vi "Internal Open.vi"(0 "navX Device":T8={"Interface"={"Protocol"=enum."SERIAL", "Update Rate (4Hz-60Hz)"=4, "navX Open TypeDef"=variant}, "Notify Packet"=refnum, "Loop VI Refnum"=refnum} {"Interface"."Update Rate (4Hz-60Hz)" min=4 max=60 step=1}) -> (1 "Interface TypeDefs":T1 {"I2CDevRef"."Device Address" format="%.0x"}, 2 "error out":errorcluster)   [LabVIEW 2014, in "navX Library v2.lvlib"]
uses:
  navX Library v2.lvlib
  TypeDefs/navX Device TypeDef.ctl
  TypeDefs/navX Protocol TypeDef.ctl
  TypeDefs/navX Notify Packet TypeDef.ctl
  TypeDefs/navX Action TypeDef.ctl
  TypeDefs/navX Interface TypeDef.ctl
  <vilib>/Rock Robotics/WPI/SerialPort/WPI_SerialPortRef.ctl
  <vilib>/Rock Robotics/WPI/I2C/WPI_I2CDevRef.ctl
  <vilib>/Rock Robotics/SystemInterfaces/Typedef/FPGA_TypedefDigitalModule.ctl
  <vilib>/Rock Robotics/SystemInterfaces/i2clib/i2c_bus.ctl
  <vilib>/Rock Robotics/WPI/SPI/WPI_SPIDevRef.ctl
  <vilib>/Rock Robotics/SystemInterfaces/spilib/spi_bus.ctl
  TypeDefs/navX Open TypeDefs/navX Serial Open TypeDef.ctl
  NI WPI/WPI_SerialPort_USB.ctl
  TypeDefs/navX Open TypeDefs/navX I2C Open TypeDef.ctl
  TypeDefs/navX Open TypeDefs/navX SPI Open TypeDef.ctl
  NI WPI/NI WPI Serial USB.lvlib
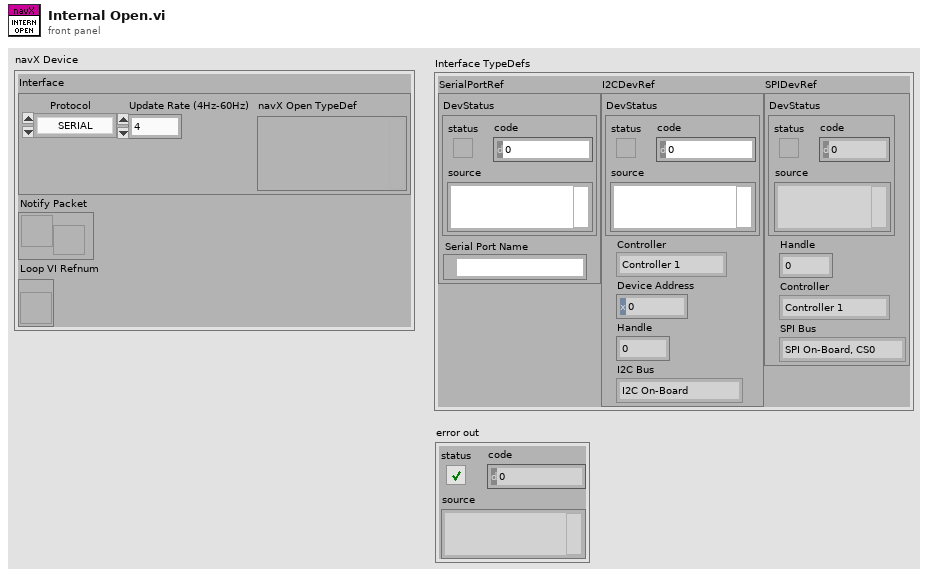
[diagram p1: front panel]
types:
  T1 = typedef "navX Library v2.lvlib/navX Interface TypeDef.ctl" = cluster{"SerialPortRef":T2, "I2CDevRef":T3, "SPIDevRef":T6}
  T2 = typedef "WPI_SerialPortRef.ctl" = cluster{"DevStatus":errorcluster, "Serial Port Name":refnum<visa-resource-name>}
  T3 = typedef "WPI_I2CDevRef.ctl" = cluster{"DevStatus":errorcluster, "Controller":T4, "Device Address":u8, "Handle":i32, "I2C Bus":T5}
  T4 = typedef "FPGA_TypedefDigitalModule.ctl" = enum16{"Controller 1"}
  T5 = typedef "i2c_bus.ctl" = enum16{"I2C On-Board", "I2C MXP", "Invalid"}
  T6 = typedef "WPI_SPIDevRef.ctl" = cluster{"DevStatus":errorcluster, "Handle":i32, "Controller":T4, "SPI Bus":T7}
  T7 = typedef "spi_bus.ctl" = enum16{"SPI On-Board, CS0", "SPI On-Board, CS1", "SPI On-Board, CS2", "SPI On-Board, CS3", "SPI MXP", "Invalid"}
  T8 = typedef "navX Library v2.lvlib/navX Device TypeDef.ctl" = cluster{"Interface":cluster{"Protocol":T9, "Update Rate (4Hz-60Hz)":u8, "navX Open TypeDef":variant}, "Notify Packet":refnum<notifier>, "Loop VI Refnum":refnum<vi>}
  T9 = typedef "navX Library v2.lvlib/navX Protocol TypeDef.ctl" = enum16{"SERIAL", "I2C", "SPI"}
  T10 = typedef "navX Library v2.lvlib/navX Serial Open TypeDef.ctl" = cluster{"Serial Port":T11, "Raw Data":bool}
  T11 = typedef "NI WPI Serial USB.lvlib/WPI_SerialPort_USB.ctl" = enum16{"Onboard RS-232", "MXP TTL", "USB"}
  T12 = typedef "navX Library v2.lvlib/navX I2C Open TypeDef.ctl" = cluster{"I2C Bus":T5}
  T13 = typedef "navX Library v2.lvlib/navX SPI Open TypeDef.ctl" = cluster{"SPI Bus":T7}
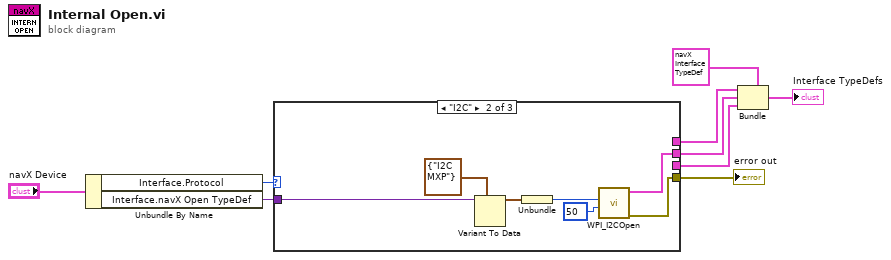
[diagram p0: block diagram]
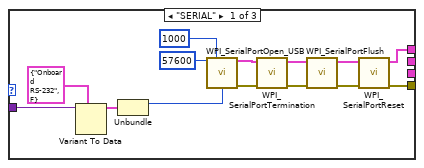
[diagram p2: hidden frame]
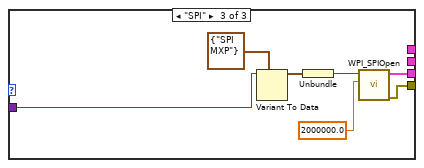
[diagram p3: hidden frame]
diagram:
  n1 = Unbundle By Name("navX Device") -> ("Interface.Protocol"=w5:T9, "Interface.navX Open TypeDef"=w4:variant)
  n2 = case shown="\"I2C\"" w5 {
    tunnel: w4 -> [w23 w29 w36]
    tunnel: [w11 _ _] -> w9
    tunnel: [w10 w25 w32] -> w3
    tunnel: [_ w24 _] -> w8
    tunnel: [_ _ w31] -> w7
    frame "SERIAL" {
      n3 = Variant To Data(type=T10 {"Serial Port"=enum."Onboard RS-232", "Raw Data"=FALSE} ("navX Serial Open"), Variant=w23) -> (data=w21:T10)  [unwired: 1 in, 1 out]
      n4 = Unbundle(w21) -> ("Serial Port"=w20:T11)  [unwired: 1 out]
      n5 = call "WPI_SerialPortOpen_USB.vi"("Baud Rate"=u32 57600, "Timeout Value (ms)"=u32 1000, "Serial Port"=w20) -> ("SerialPortRef"=w13:T2, "error out"=w12:errorcluster)  [unwired: 11 in]
      n6 = call <vilib>:"WPI_SerialPortTermination.vi"("error in (no error)"=w12, "SerialPortRef"=w13) -> ("error out"=w17:errorcluster, "SerialPortRef"=w16:T2)  [unwired: 8 in]
      n7 = call <vilib>:"WPI_SerialPortFlush.vi"("error in (no error)"=w17, "SerialPortRef"=w16) -> ("error out"=w14:errorcluster, "SerialPortRef"=w15:T2)  [unwired: 8 in]
      n8 = call <vilib>:"WPI_SerialPortReset.vi"("error in (no error)"=w14, "SerialPortRef"=w15) -> ("error out"=w10:errorcluster, "SerialPortRef"=w11:T2)  [unwired: 8 in]
    }
    frame "I2C" {
      n9 = Variant To Data(type=T12 {"I2C Bus"=enum."I2C MXP"} ("navX I2C Open"), Variant=w29) -> (data=w30:T12)  [unwired: 1 in, 1 out]
      n10 = Unbundle(w30) -> ("I2C Bus"=w27:T5)
      n11 = call <vilib>:"WPI_I2COpen.vi"("Device Address"=u8 50, "I2C Bus"=w27) -> ("error out"=w25:errorcluster, "I2CDevRef"=w24:T3)  [unwired: 8 in]
    }
    frame "SPI" {
      n12 = Variant To Data(type=T13 {"SPI Bus"=enum."SPI MXP"} ("navX SPI Open"), Variant=w36) -> (data=w37:T13)  [unwired: 1 in, 1 out]
      n13 = Unbundle(w37) -> ("SPI Bus"=w34:T7)
      n14 = call <vilib>:"WPI_SPIOpen.vi"("Clock Rate (Hz)"=2000000.0, "SPI Bus"=w34) -> ("error out"=w32:errorcluster, "SPIDevRef"=w31:T6)  [unwired: 8 in]
    }
  }
  "error out" <- w3
  n15 = Bundle(cluster=T1 {"SerialPortRef"={"DevStatus"={"status"=FALSE, "code"=0, "source"=""}, "Serial Port Name"=""}, "I2CDevRef"={"DevStatus"={"status"=FALSE, "code"=0, "source"=""}, "Controller"=enum."Controller 1", "Device Address"=0, "Handle"=0, "I2C Bus"=enum."I2C On-Board"}, "SPIDevRef"={"DevStatus"={"status"=FALSE, "code"=0, "source"=""}, "Handle"=0, "Controller"=enum."Controller 1", "SPI Bus"=enum."SPI On-Board, CS0"}} ("Interface TypeDefs"), "SerialPortRef"=w9, "I2CDevRef"=w8, "SPIDevRef"=w7) -> (→"Interface TypeDefs":T1)
